vi "Test Method Result Execution Time.vi"(8 "error in (no error)":errorcluster, 11 "Pass Assertion Test In":refnum<class "Method Result Test.lvclass">) -> (0 "error out":errorcluster, 3 "Pass Assertion Test Out":refnum<class "Method Result Test.lvclass">)   [LabVIEW 2020, in "LUnit Tests.lvlib" / "Method Result Test.lvclass"]
uses:
  Method Result Test.lvclass
  C:/Program Files (x86)/National Instruments/LabVIEW 2020/vi.lib/Asteme/LUnit/Test Case.lvclass
  source/Framework/Result Classes/Method Result/Method Result.lvclass/Method Result.ctl
  <vilib>/Asteme/LUnit/Test Case.lvclass/Test Case.ctl
  <vilib>/Asteme/LUnit/LUnit Assertion Result.lvclass/LUnit Assertion Result.ctl
  <vilib>/Asteme/LUnit/LUnit Test Case Result.lvclass/LUnit Test Case Result.ctl
  <vilib>/Asteme/LUnit/LUnit Method Result.lvclass/LUnit Method Result.ctl
  <vilib>/Asteme/LUnit/Set Assertion Type.vi
  <vilib>/Asteme/LUnit/Palette/Pass.vi
  <vilib>/Asteme/LUnit/Palette/Fail.vi
  <vilib>/Asteme/LUnit/LUnit Write Assertion Type.vi
  <vilib>/Asteme/LUnit/Add test result.vi
  <vilib>/Asteme/LUnit/LUnit Write Passed.vi
  <vilib>/Asteme/LUnit/LUnit Write Message.vi
  <vilib>/Asteme/LUnit/LUnit Write Description.vi
  <vilib>/Asteme/LUnit/LUnit Record Assertion Result.vi
  <vilib>/Asteme/LUnit/LUnit Aggregate Assertion Results.vi
  <vilib>/Asteme/LUnit/Assertion Result/LUnit Read Status.vi
  <vilib>/Asteme/LUnit/LUnit Read Message.vi
  <vilib>/Asteme/LUnit/LUnit Read Description.vi
  <vilib>/Asteme/LUnit/Method Result/LUnit Merge Status.vi
  <vilib>/Asteme/LUnit/LUnit Concatenate result strings.vi
  <vilib>/Asteme/LUnit/LUnit Assertion Result.lvclass
  source/Framework/Result Classes/Method Result/Method Result.lvclass
  <vilib>/Asteme/LUnit/Test Case.lvclass
  C:/Users/anton/Documents/GitHub/LUnit/tests/Framework Test/Assertion Test/Method Result Test.lvclass
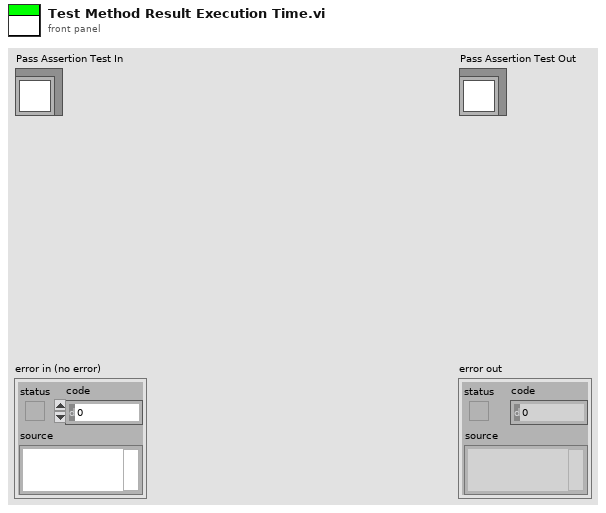
[diagram p1: front panel]
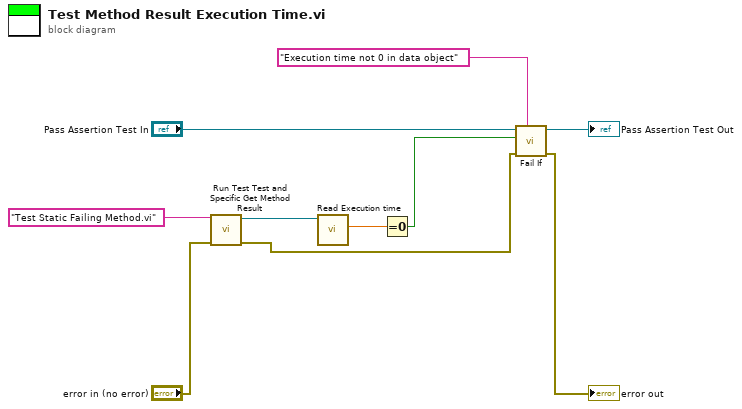
[diagram p0: block diagram]
diagram:
  n1 = call "Run Test Test and Specific Get Method Result.vi"("error in (no error)"="error in (no error)", "Method of Interest"="Test Static Failing Method.vi") -> ("error out"=w1:errorcluster, "Method Result out"=w4:refnum<class "Method Result.lvclass">)  [unwired: 8 in]
  n2 = call "Read Execution time.vi"("Method Result In"=w4) -> ("Execution time"=w6:dbl)  [unwired: 8 in, 2 out]
  n3 = Equal To 0?(x=w6) -> (x = 0?=w5:bool)
  n4 = call <vilib>:"Fail If.vi"("Description"="Execution time not 0 in data object", "error in (no error)"=w1, "Fail?"=w5, "LUnit Test Case In"="Pass Assertion Test In") -> ("error out"=→"error out":errorcluster, "LUnit Test Case Out"=→"Pass Assertion Test Out":refnum<class "Method Result Test.lvclass">)  [unwired: 6 in]
